vi "Sample8742UIyes.vi"() -> ()   [LabVIEW 2021]
uses:
  Global Variablesyes.vi
panel:
  out "error out":errorcluster
  out "In Motion":bool
  out "Status:":string
  out "Current Position:":string
  in  "Stop":bool
  in  "Go":bool
  in  "Relative Move:":string
  in  "Selected Motor:":string(combo)
  in  "Selected Controller:":string(combo)
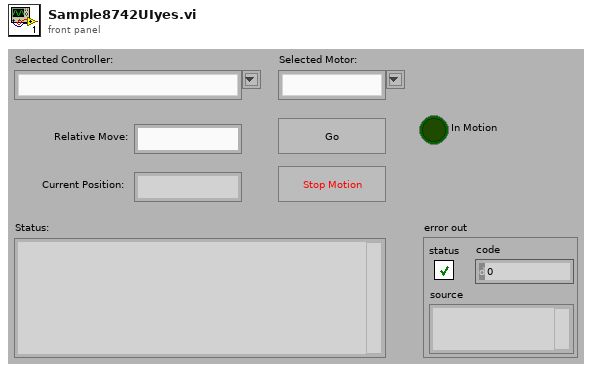
[diagram p1: front panel]
types:
  T1 = cluster{"Selected Controller:":refnum<vi>, "Selected Motor:":refnum<vi>, "Relative Move:":refnum<vi>, "Current Position:":refnum<vi>, "Go":refnum<vi>, "Stop":refnum<vi>}
  T2 = cluster{"DeviceKey":string, "Device Address":i32, "Controller Name":string}[]
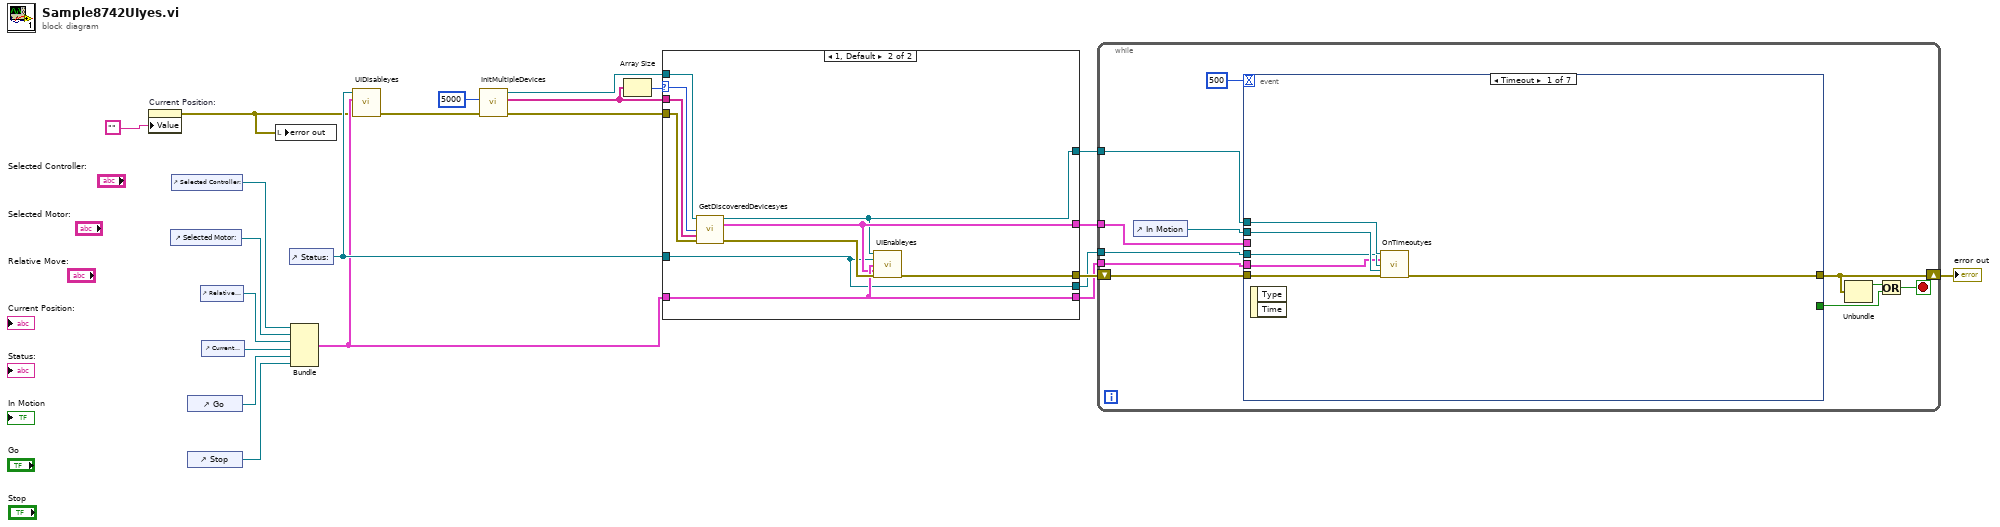
[diagram p0: block diagram]
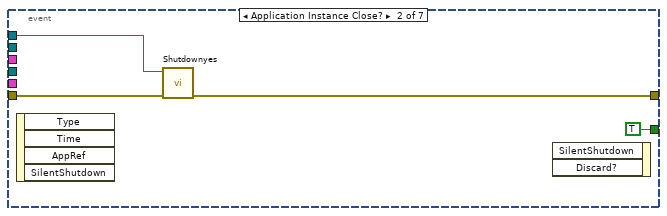
[diagram p2: hidden frame]
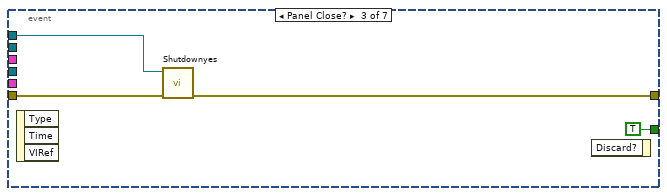
[diagram p3: hidden frame]
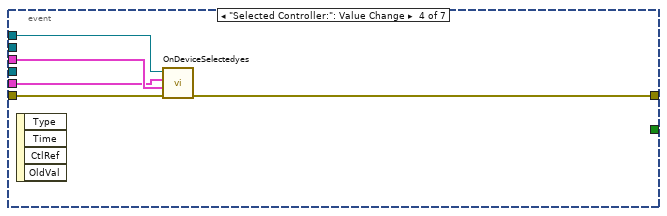
[diagram p4: hidden frame]
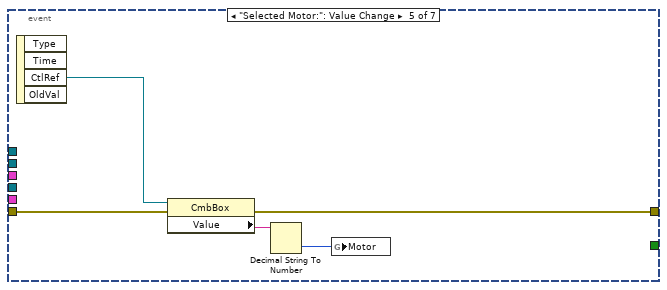
[diagram p5: hidden frame]
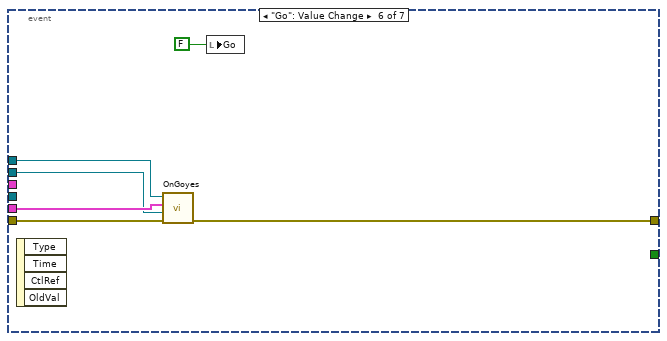
[diagram p6: hidden frame]
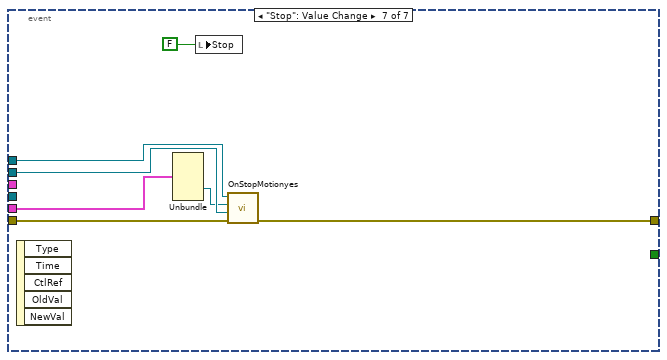
[diagram p7: hidden frame]
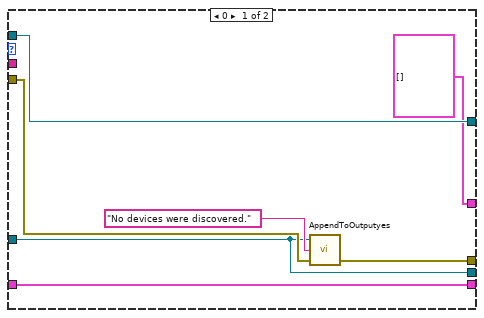
[diagram p8: hidden frame]
diagram:
  n1 = property on="Current Position:" class="Str"("Value"="") -> (error out=w1:errorcluster)  [unwired: 2 in, 1 out]
  n2 = control-ref of="Selected Motor:"() -> (w22:refnum<vi>)
  n3 = control-ref of="Selected Controller:"() -> (w14:refnum<vi>)
  n4 = control-ref of="Go"() -> (w4:refnum<vi>)
  n5 = control-ref of="Stop"() -> (w5:refnum<vi>)
  n6 = control-ref of="Relative Move:"() -> (w21:refnum<vi>)
  n7 = control-ref of="Current Position:"() -> (w3:refnum<vi>)
  n8 = local write "error out"(w1) -> ()
  n9 = control-ref of="Status:"() -> (w13:refnum<vi>)
  n10 = Bundle("Selected Controller:"=w14, "Selected Motor:"=w22, "Relative Move:"=w21, "Current Position:"=w3, "Go"=w4, "Stop"=w5) -> (w9:T1)  [unwired: 1 in]
  n11 = call "UIDisableyes.vi"("error in (no error)"=w1, "UI"=w9, "Status:"=w13) -> ("error out"=w20:errorcluster)  [unwired: 8 in]
  n12 = call "InitMultipleDevices.vi"("error in (no error)"=w20, "msecDelayForDiscovery"=5000) -> ("error out"=w17:errorcluster, "DeviceKey List Out"=w15:string[], "CmdLib Out"=w16:refnum<k24>)  [unwired: 3 in]
  n13 = Array Size(array=w15) -> (size(s)=w18:i32)
  n14 = case shown="1, Default" w18 {
    selector: w18 -> [_ w35]
    tunnel: w13 -> [w23 w30]
    tunnel: w17 -> [w28 w38]
    tunnel: w16 -> [w26 w39]
    tunnel: w15 -> [_ w37]
    tunnel: [w27 w34] -> w12
    tunnel: [w26 w31] -> w11
    tunnel: w9 -> [w25 w33]
    tunnel: [w25 w33] -> w7
    tunnel: [T2 [] ("Device Array") w32] -> w6
    tunnel: [w23 w30] -> w2
    frame 0 {
      n15 = call "AppendToOutputyes.vi"("error in"=w28, "Input String"="No devices were discovered.", "Output Refnum In"=w23) -> ("error out"=w27:errorcluster)  [unwired: 1 in, 1 out]
    }
    frame 1, Default {
      n16 = call "GetDiscoveredDevicesyes.vi"("CmdLib In"=w39, "Master Count"=w35, "DeviceKey List"=w37, "error in"=w38) -> ("CmdLib Out"=w31:refnum<k24>, "Device Array"=w32:T2, "error out"=w36:errorcluster)  [unwired: 9 in]
      n17 = call "UIEnableyes.vi"("CmdLib In"=w31, "Status:"=w30, "UI"=w33, "Device Array"=w32, "error in"=w36) -> ("error out"=w34:errorcluster)  [unwired: 10 in]
    }
  }
  n18 = while {
    tunnel: w11 -> [w49]
    tunnel: w7 -> [w48]
    tunnel: w6 -> [w47]
    shift-right: [w44] -> w8
    shift-left: w12 -> [w50]
    tunnel: w2 -> [w45]
    stop <- w43 stop-if-true
    n19 = control-ref of="In Motion"() -> (w40:refnum<vi>)
    n20 = event shown="[0] Timeout" {
      selector: _ -> [_ _ _ _ _ _ _]
      dyn-events: _ -> [_ _ _ _ _ _ _]
      timeout: 500 -> [_ _ _ _ _ _ _]
      tunnel: w50 -> [w56 w60 w63 w69 w72 w80 w86]
      tunnel: w49 -> [w53 w59 w64 w65 _ w78 w85]
      tunnel: [_ TRUE TRUE _ _ _ _] -> w41
      tunnel: [w55 w57 w61 w68 w71 w75 w83] -> w44
      tunnel: w48 -> [w51 _ _ w66 _ w79 w82]
      tunnel: w47 -> [_ _ _ w67 _ _ _]
      tunnel: w45 -> [w52 _ _ _ _ _ _]
      tunnel: w40 -> [w54 _ _ _ _ w77 w87]
      event Timeout {
        n21 = event-data() -> ()  [unwired: 1 in, 2 out]
        n22 = call "OnTimeoutyes.vi"("CmdLib In"=w53, "UI"=w51, "Status:"=w52, "In Motion"=w54, "error in"=w56) -> ("error out"=w55:errorcluster)  [unwired: 10 in]
      }
      event Application Instance Close? {
        n23 = event-data() -> ()  [unwired: 1 in, 4 out]
        n24 = call "Shutdownyes.vi"("error in (no error)"=w60, "CmdLib In"=w59) -> ("error out"=w57:errorcluster)  [unwired: 4 in, 1 out]
        n25 = event-data() -> ()  [unwired: 3 in, 1 out]
      }
      event Panel Close? {
        n26 = event-data() -> ()  [unwired: 1 in, 3 out]
        n27 = call "Shutdownyes.vi"("error in (no error)"=w63, "CmdLib In"=w64) -> ("error out"=w61:errorcluster)  [unwired: 4 in, 1 out]
        n28 = event-data() -> ()  [unwired: 2 in, 1 out]
      }
      event "Selected Controller:": Value Change {
        n29 = event-data() -> ()  [unwired: 1 in, 4 out]
        n30 = call "OnDeviceSelectedyes.vi"("error in"=w69, "Device Array"=w67, "UI"=w66, "CmdLib In"=w65) -> ("error out"=w68:errorcluster)  [unwired: 7 in]
      }
      event "Selected Motor:": Value Change {
        n31 = event-data() -> ("CtlRef"=w70:refnum<vi>)  [unwired: 1 in, 3 out]
        n32 = property class="CmbBox"(reference=w70, error in=w72) -> (error out=w71:errorcluster, "Value"=w74:string)  [unwired: 1 out]
        n33 = Decimal String To Number(string=w74) -> (number=w73:i32)  [unwired: 2 in, 1 out]
        n34 = global write "Global Variablesyes.vi" "Motor"(w73) -> ()
      }
      event "Go": Value Change {
        n35 = event-data() -> ()  [unwired: 1 in, 4 out]
        n36 = call "OnGoyes.vi"("error in"=w80, "In Motion"=w77, "UI"=w79, "CmdLib Out"=w78) -> ("error out"=w75:errorcluster)  [unwired: 7 in]
        n37 = local write "Go"(FALSE ("Go")) -> ()
      }
      event "Stop": Value Change {
        n38 = event-data() -> ()  [unwired: 1 in, 5 out]
        n39 = Unbundle(w82) -> ("Go"=w81:refnum<vi>)  [unwired: 5 out]
        n40 = local write "Stop"(FALSE ("Stop")) -> ()
        n41 = call "OnStopMotionyes.vi"("error in"=w86, "In Motion"=w87, "Go"=w81, "CmdLib In"=w85) -> ("error out"=w83:errorcluster)  [unwired: 7 in]
      }
    }
    n42 = Unbundle(w44) -> ("status"=w42:bool)  [unwired: 2 out]
    n43 = Or(x=w42, y=w41) -> (x .or. y?=w43:bool)
  }
  "error out" <- w8
